vi "myRIO_Brig_RT__Case_Exp_State_initBlock.vi"(8 "input_spout":enum16{"Left", "Right"}(ring), 10 "input_dataExp":u16[](array[numeric]), 11 "input_dataCurrent":u16[](array[numeric])) -> (0 "output_spout":enum16{"Left", "Right"}(ring), 1 "output_state":T1=enum."initTrial", 2 "output_dataExp":u16[](array[numeric]), 3 "output_dataCurrent":u16[](array[numeric]), 4 "output_TpB_target":u16)   [LabVIEW 2014]
uses:
  myRIO_BRig_RT__Case_Exp_stateList.ctl
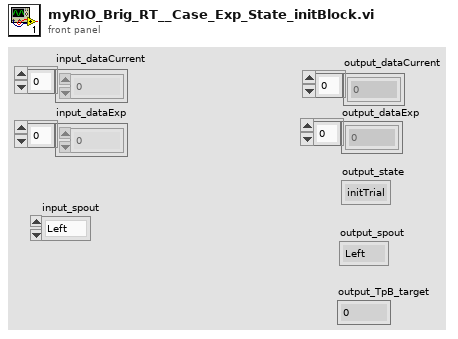
[diagram p1: front panel]
types:
  T1 = typedef "myRIO_BRig_RT__Case_Exp_stateList.ctl" = enum16{"Start1", "Start2", "Start3", "saveSettings1", "saveSettings2", "saveSettings3", "saveSettings4", "saveSettings_LC_ENL_l1", "saveSettings_LC_ENL_l2", "saveSettings_LC_Cue_l1", "saveSettings_LC_Cue_l2", "saveSettings6_LC_l1_Other", "SaveSettings6_LC_l2_Other", "setSettings_Audio", "setSettings_Laser", "initBlock_pre", "initBlock", "initBlock2", "initBlock_post", "initTrial_pre", "initTrial", "initTrial2", "initTrial3", "initTrial4", "initTrial_LC_ENL1", "initTrial_LC_Cue1", "initTrial_LC_Cue1_2", "initTrial_LC_Sel", "initTrial_post", "ENL1_pre", "ENL1", "ENL1_post", "ENL1Penalty_pre", "ENL1Penalty", "ENL2_pre", "ENL2", "ENL2Penalty_pre", "ENL2Penalty", "Cue1_pre", "Cue1", "Cue1_post", "Cue1Penalty_pre", "Cue1Penalty", "Cue2_pre", "Cue2", "Cue2Penalty_pre", "Cue2Penalty", "Selection_pre", "Selection", "Select_post", "SelectReward_pre", "SelectReward", "SelectRewardPost_pre", "SelectRewardPost", "SelectWrong_pre", "SelectWrong", "SelectWrong_post", "SelectTimeout_pre", "SelectTimeout", "SelectTimeout_post", "endTrial_pre", "endTrial1", "endTrial2", "endTrial3", "endTrial_post", "endBlock_pre", "endBlock", "endBlock_post", "endExp", "commConnect", "commUpload_pre", "commUpload_dataBlock", "commUpload_dataCurrent", "commUpload_dataExp", "commUpload_dataLC", "commUpload_dataTrial", "commUpload_post", "saveData_pre", "saveData_dataBlock", "saveData_dataCurrent", "saveData_dataExp", "saveData_dataLC", "saveData_dataTrial", "saveData_post", "empty_endBlock1", "empty_endBlock2", "empty_endTrial1", "empty_endTrial2", "empty_endTrial3", "empty_endTrial4", "empty_endTrial5", "dummyState", "dummyState_endBlock"}
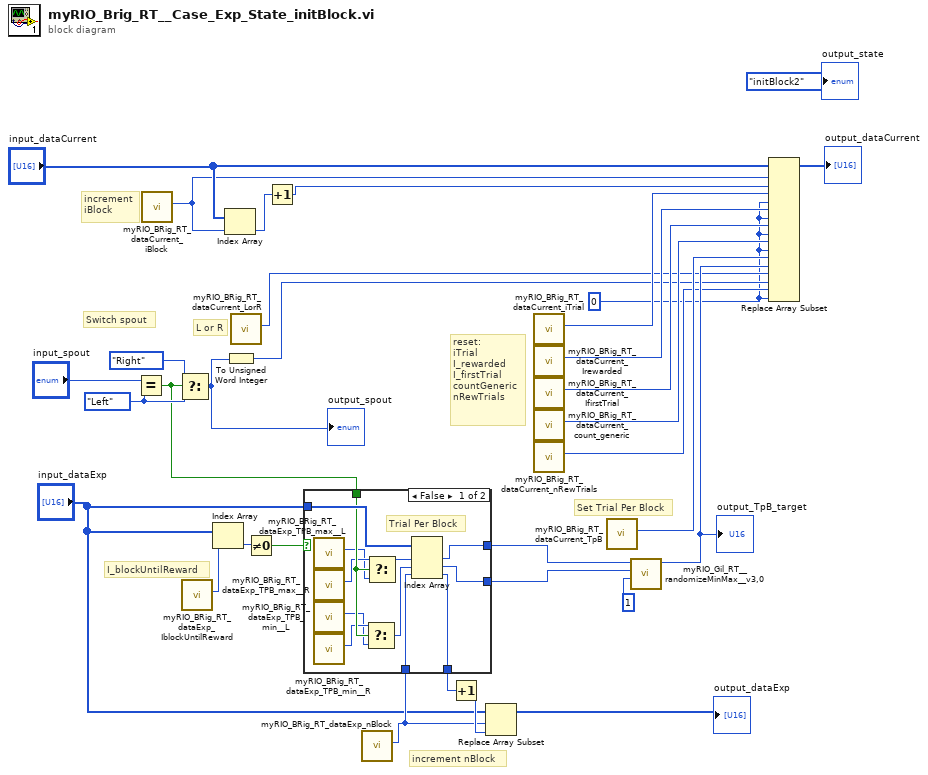
[diagram p0: block diagram]
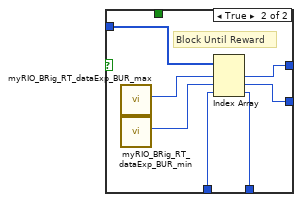
[diagram p2: hidden frame]
diagram:
  w2 = u16 0
  w32 = enum16{"Left", "Right"}."Left"
  # "L or R"
  # "I_blockUntilReward"
  # "increment nBlock"
  # "reset:\niTrial\nI_rewarded\nI_firstTrial\ncountGeneric\nnRewTrials"
  # "increment\niBlock"
  # "Set Trial Per Block"
  # "Switch spout"
  n1 = Equal?(x="input_spout", y=w32) -> (x = y?=w1:bool)
  n2 = call "myRIO_BRig_RT_dataCurrent_iBlock.vi"() -> ("output_iBlock"=w26:i32)  [unwired: 11 in]
  n3 = Select(t=enum16{"Left", "Right"}."Right", s=w1, f=w32) -> (s? t:f=w4:enum16{"Left", "Right"})
  "output_spout" <- w4
  n4 = call "myRIO_BRig_RT_dataExp_IblockUntilReward.vi"() -> ("output_I_blockUntilReward"=w13:i32)  [unwired: 11 in]
  n5 = Index Array(array="input_dataExp", index=w13) -> (element=w12:u16)
  n6 = Index Array(array="input_dataCurrent", index=w26) -> (element=w27:u16)
  n7 = To Unsigned Word Integer(number=w4) -> (unsigned 16bit integer=w5:u16)
  n8 = call "myRIO_BRig_RT_dataCurrent_LorR.vi"() -> ("output_LorR"=w7:i32)  [unwired: 11 in]
  n9 = Not Equal To 0?(x=w12) -> (x != 0?=w11:bool)
  n10 = Increment(x=w27) -> (x+1=w25:u16)
  n11 = call "myRIO_BRig_RT_dataExp_nBlock.vi"() -> ("output_nBlock"=w19:i32)  [unwired: 11 in]
  n12 = case shown="False" w11 {
    tunnel: w19 -> [w42 w49]
    tunnel: [w41 w48] -> w18
    tunnel: "input_dataExp" -> [w44 w47]
    tunnel: [w39 w46] -> w9
    tunnel: [w40 w45] -> w8
    tunnel: w1 -> [w43 _]
    frame False {
      # "Trial Per Block"
      n13 = call "myRIO_BRig_RT_dataExp_TPB_max__L.vi"() -> ("output_TPB_max__L"=w33:i32)  [unwired: 11 in]
      n14 = call "myRIO_BRig_RT_dataExp_TPB_max__R.vi"() -> ("output_TPB_max__R"=w34:i32)  [unwired: 11 in]
      n15 = call "myRIO_BRig_RT_dataExp_TPB_min__L.vi"() -> ("output_TPB_min__L"=w35:i32)  [unwired: 11 in]
      n16 = call "myRIO_BRig_RT_dataExp_TPB_min__R.vi"() -> ("output_TPB_min__R"=w36:i32)  [unwired: 11 in]
      n17 = Select(t=w36, s=w43, f=w35) -> (s? t:f=w37:i32)
      n18 = Select(t=w34, s=w43, f=w33) -> (s? t:f=w38:i32)
      n19 = Index Array(array=w44, index #1=w38, index #2=w37, index #3=w42) -> (element #1=w39:u16, element #2=w40:u16, element #3=w41:u16)
    }
    frame True {
      # "Block Until Reward"
      n20 = call "myRIO_BRig_RT_dataExp_BUR_max.vi"() -> ("output_BUR_max"=w51:i32)  [unwired: 11 in]
      n21 = call "myRIO_BRig_RT_dataExp_BUR_min.vi"() -> ("output_BUR_min"=w50:i32)  [unwired: 11 in]
      n22 = Index Array(array=w47, index #1=w51, index #2=w50, index #3=w49) -> (element #1=w46:u16, element #2=w45:u16, element #3=w48:u16)
    }
  }
  n23 = Increment(x=w18) -> (x+1=w21:u16)
  n24 = Replace Array Subset(array="input_dataExp", new element=w21, index=w19) -> (→"output_dataExp":u16[])
  n25 = call "myRIO_BRig_RT_dataCurrent_iTrial.vi"() -> ("output_iTrial"=w24:i32)  [unwired: 11 in]
  n26 = call "myRIO_BRig_RT_dataCurrent_Irewarded.vi"() -> ("output_I_rewarded"=w23:i32)  [unwired: 11 in]
  n27 = call "myRIO_BRig_RT_dataCurrent_IfirstTrial.vi"() -> ("output_I_firstTrial"=w22:i32)  [unwired: 11 in]
  n28 = call "myRIO_BRig_RT_dataCurrent_count_generic.vi"() -> ("output_count_generic"=w14:i32)  [unwired: 11 in]
  n29 = call "myRIO_BRig_RT_dataCurrent_nRewTrials.vi"() -> ("output_nRewTrials"=w3:i32)  [unwired: 11 in]
  n30 = call "myRIO_BRig_RT_dataCurrent_TpB.vi"() -> ("output_TpB"=w15:i32)  [unwired: 11 in]
  n31 = call "myRIO_Gil_RT__randomizeMinMax__v3,0.vi"("Input_Increment"=u16 1, "Input_Min"=w8, "Input_Max"=w9) -> ("Output"=w16:u16)  [unwired: 8 in]
  "output_TpB_target" <- w16
  n32 = Replace Array Subset(array="input_dataCurrent", new element #1=w25, index #1=w26, new element #2=w2, index #2=w24, new element #3=w2, index #3=w23, new element #4=w2, index #4=w22, new element #5=w2, index #5=w14, new element #6=w16, index #6=w15, new element #7=w5, index #7=w7, new element #8=w2, index #8=w3) -> (→"output_dataCurrent":u16[])
  "output_state" <- myRIO_BRig_RT__Case_Exp_stateList."initBlock2" ("Enum")
